vi "Temperature Limit.vi"() -> ()   [LabVIEW 2014]
doc: "This VI simulates the acquisition of temperature, graphs the temperature, and notifies the user if the temperature is over the limit."
uses:
  <vilib>/ErrorRing/Error Ring.xnode
panel:
  in  "Start":bool
  in  "Delta t (ms)":i32(slide)=400 scale=50.0..500.0
  in  "Stop":bool
  in  "High Limit":dbl=28.0 format="%.2f"
  out "Temperature":cluster{"Temperature":dbl, "High Limit":dbl}(graph)={"Temperature"=85.88749999999999, "High Limit"=80.0}
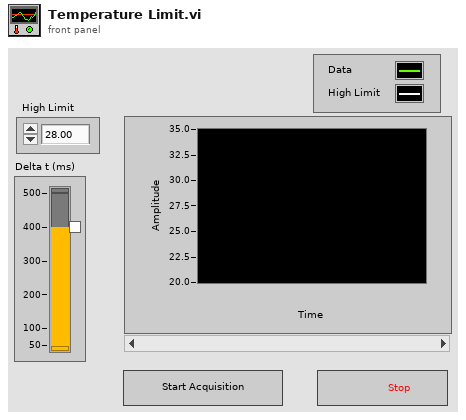
[diagram p1: front panel]
types:
  T1 = cluster{"Temperature Value":dbl, "High Limit":dbl}
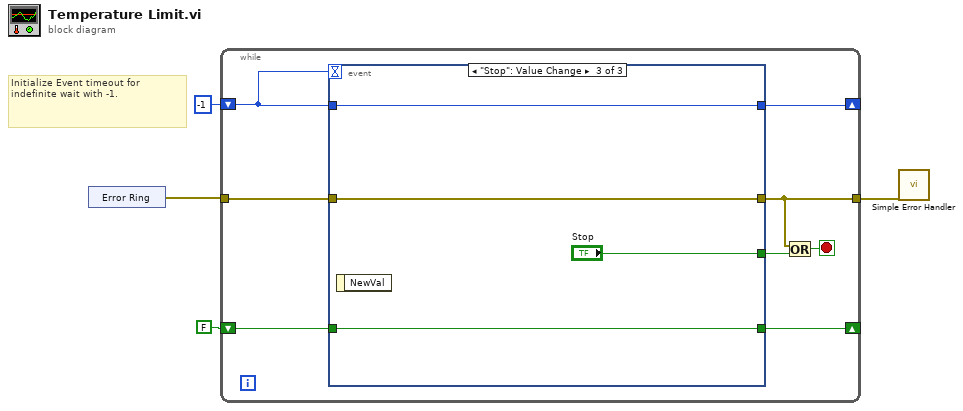
[diagram p0: block diagram]
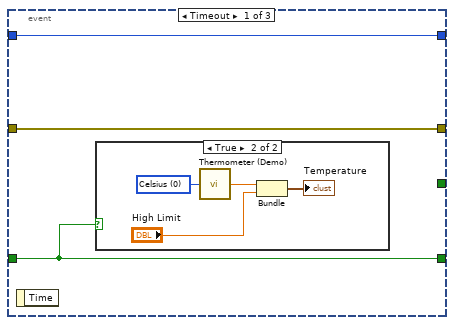
[diagram p2: hidden frame]
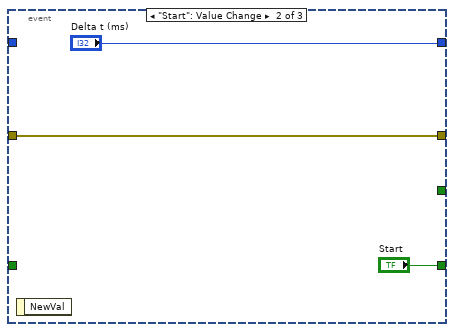
[diagram p4: hidden frame]
diagram:
  # "Initialize Event timeout for indefinite wait with -1."
  n1 = xnode "Error Ring"() -> ("error out"=w1:errorcluster)
  n2 = while {
    tunnel: w1 -> [w12]
    tunnel: [w10] -> w3
    shift-right: [w8] -> _
    shift-left: FALSE ("Start") -> [w7]
    shift-right: [w6] -> _
    shift-left: -1 ("Delta t (ms)") -> [w5]
    stop <- w11 stop-if-true
    n3 = event shown="[2] \"Stop\": Value Change" {
      selector: _ -> [_ _ _]
      dyn-events: _ -> [_ _ _]
      timeout: w5 -> [_ _ _]
      tunnel: [_ _ "Stop"] -> w9
      tunnel: w12 -> [w15 w20 w25]
      tunnel: [w15 w20 w25] -> w10
      tunnel: [w13 "Start" w24] -> w8
      tunnel: w7 -> [w13 _ w24]
      tunnel: [w14 "Delta t (ms)" w23] -> w6
      tunnel: w5 -> [w14 _ w23]
      event Timeout {
        n4 = event-data() -> ()  [unwired: 1 in, 1 out]
        n5 = case shown="True" w13 {
          frame False {
          }
          frame True {
            w16 = u16 0 items=["Celsius", "Fahrenheit"] ("Units (0: Celsius)")
            n6 = call "Thermometer (Demo).vi"("Units (0: Celsius)"=w16) -> ("Temperature Value"=w17:dbl)
            n7 = Bundle("Temperature Value"=w17, "High Limit"="High Limit") -> (→"Temperature":T1)  [unwired: 1 in]
          }
        }
      }
      event "Start": Value Change {
        n8 = event-data() -> ()  [unwired: 1 in, 1 out]
      }
      event "Stop": Value Change {
        n9 = event-data() -> ()  [unwired: 1 in, 1 out]
      }
    }
    n10 = Or(x=w10, y=w9) -> (x .or. y?=w11:bool)
  }
  n11 = call <vilib>:"Simple Error Handler.vi"("error in (no error)"=w3) -> ()  [unwired: 4 in, 5 out]
